vi "AG34980A_Configure_4-Wire_Resistance.vi"(0 "VISA resource name":refnum<visa-resource-name>, 5 "Range (7:Auto)":T2(ring)=enum."Auto", 7 "Resolution (5:Default)":T1(ring)=enum."Default", 11 "error in (no error)":errorcluster, 12 "Offset Compensation (F:Off)":bool) -> (4 "VISA resource name out":refnum<visa-resource-name>, 15 "error out":errorcluster)   [LabVIEW 2022 SP3, in "DMM_Keysight_34980A.lvlib" / "DMM_Keysight_34980A.lvclass"]
doc: "This VI allows you to specify various settings for performing 4-wire resistance measurements. You can independently control the range, resolution, autozero mode, and offset compensation settings."
uses:
  DMM_Keysight_34980A.lvclass
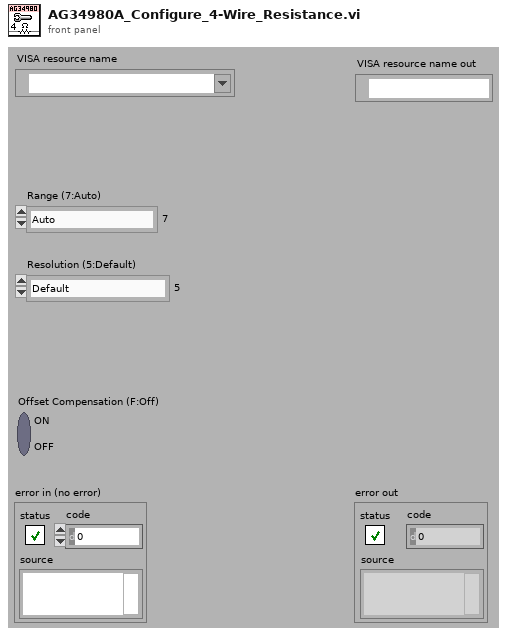
[diagram p1: front panel]
types:
  T1 = enum16{"4 1/2", "5 1/2", "6 1/2", "Least", "Highest", "Default"}
  T2 = enum16{"100 Ohm", "1 kOhm", "10 kOhm", "100 kOhm", "1 MOhm", "10 MOhm", "100 MOhm", "Auto", "Minimum", "Maximum", "Default"}
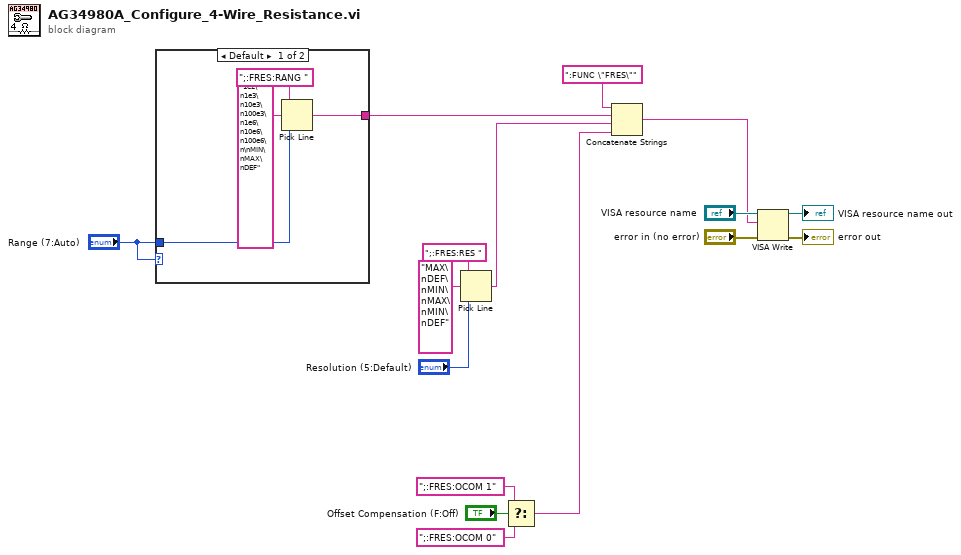
[diagram p0: block diagram]
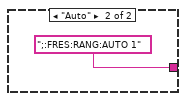
[diagram p2: hidden frame]
diagram:
  n1 = case shown="Default" "Range (7:Auto)" {
    tunnel: "Range (7:Auto)" -> [w19 _]
    tunnel: [w18 ";:FRES:RANG:AUTO 1"] -> w16
    frame Default {
      n2 = Pick Line(string ("")=";:FRES:RANG ", multi-line string="1e2\n1e3\n10e3\n100e3\n1e6\n10e6\n100e6\n\nMIN\nMAX\nDEF", line index=w19) -> (output string=w18:string)
    }
    frame "Auto" {
    }
  }
  n3 = Pick Line(string ("")=";:FRES:RES ", multi-line string="MAX\nDEF\nMIN\nMAX\nMIN\nDEF", line index="Resolution (5:Default)") -> (output string=w1:string)
  n4 = Select(t=";:FRES:OCOM 1", s="Offset Compensation (F:Off)", f=";:FRES:OCOM 0") -> (s? t:f=w7:string)
  n5 = Concatenate Strings(":FUNC \"FRES\"", w16, w1, w7) -> (w11:string)
  n6 = VISA Write(VISA resource name="VISA resource name", write buffer=w11, error in (no error)="error in (no error)") -> (VISA resource name out=→"VISA resource name out":refnum<visa-resource-name>, error out=→"error out":errorcluster)  [unwired: 1 out]
